vi "Configurar.vi"(8 "error in (no error)":errorcluster, 11 "Webcam in":refnum<class "Webcam.lvclass">) -> (0 "error out":errorcluster, 3 "Webcam out":refnum<class "Webcam.lvclass">)   [LabVIEW 2020, in "Webcam.lvclass"]
uses:
  Webcam.lvclass
  Webcam.lvclass/Webcam.ctl
  Write Session Out.vi
  Abstracta/Camara/Camara.lvclass
  <vilib>/vision/driver/NI_Vision_Acquisition_Software.lvlib
panel:
  in  "Confirm":bool
  in  "Combo Box":string(combo)
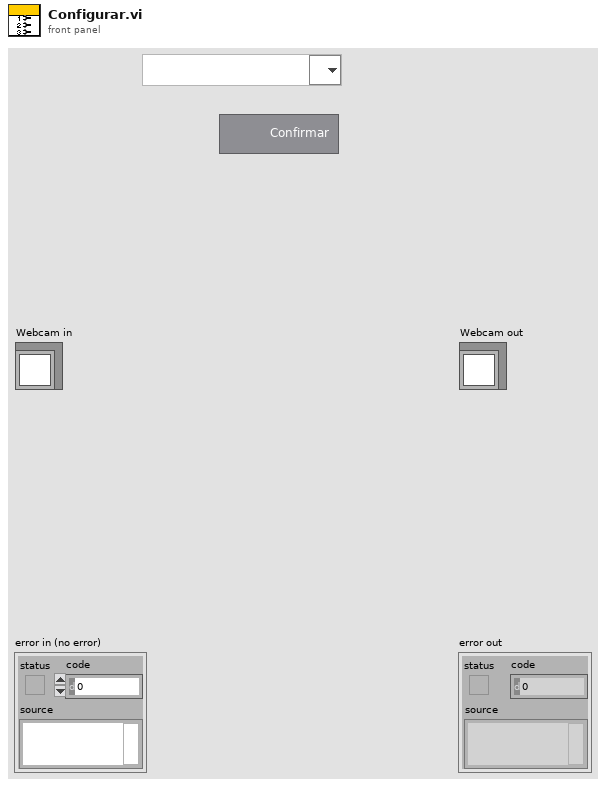
[diagram p1: front panel]
types:
  T1 = cluster{"Type":u32, "Version":u32, "Flags":u32, "SerialNumberHigh":u32, "SerialNumberLow":u32, "BusType":u32, "InterfaceName":string, "VendorName":string, "ModelName":string, "CameraFileName":string, "CameraAttributeURL":string}[]
  T2 = typedef "IMAQdx.ctl" = refnum<k21>
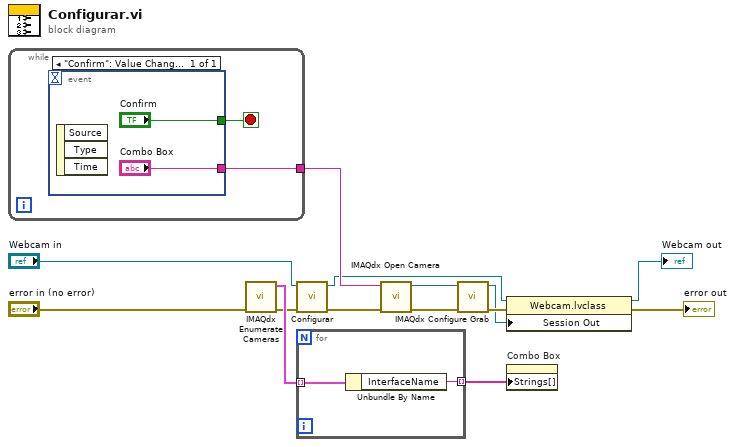
[diagram p0: block diagram]
diagram:
  n1 = while {
    tunnel: [w16] -> w11
    stop <- w15 stop-if-true
    n2 = event shown="[0] \"Confirm\": Value Change" {
      selector: _ -> [_]
      dyn-events: _ -> [_]
      timeout: _ -> [_]
      tunnel: ["Combo Box"] -> w16
      tunnel: ["Confirm"] -> w15
      event "Confirm": Value Change {
        n3 = event-data() -> ()  [unwired: 1 in, 3 out]
      }
    }
  }
  n4 = call <vilib>:"IMAQdx Enumerate Cameras.vi"("error in"="error in (no error)") -> ("error out"=w2:errorcluster, "Camera Information Array"=w13:T1)  [unwired: 9 in]
  n5 = call-parent "Configurar.vi"("error in (no error)"=w2, "Camara in"="Webcam in") -> ("error out"=w8:errorcluster, "Camara out"=w5:refnum<class "Webcam.lvclass">)  [unwired: 8 in]
  n6 = for {
    tunnel: w13 -> [w20] mode=indexing
    tunnel: [w19] -> w12 mode=indexing
    n7 = Unbundle By Name(w20) -> ("InterfaceName"=w19:string)
  }
  n8 = call <vilib>:"IMAQdx Open Camera.vi"("error in"=w8, "Session In"=w11) -> ("error out"=w9:errorcluster, "Session Out"=w10:T2)  [unwired: 8 in]
  n9 = call <vilib>:"IMAQdx Configure Grab.vi"("error in"=w9, "Session In"=w10) -> ("error out"=w7:errorcluster, "Session Out"=w3:T2)  [unwired: 8 in]
  n10 = property class="Webcam.lvclass"(reference=w5, error in=w7, "Session Out"=w3) -> (reference out=→"Webcam out":refnum<class "Webcam.lvclass">, error out=→"error out":errorcluster)
  n11 = property on="Combo Box" class="CmbBox"("Strings[]"=w12) -> ()  [unwired: 2 in, 2 out]
